vi "Release.vi"(8 "error in (no error)":errorcluster, 11 "Panel Registry in":refnum<class "Panel Registry.lvclass">) -> (0 "error out":errorcluster)   [LabVIEW 2023, in "Panel Actor.lvlib" / "Panel.lvlib" / "Panel Registry.lvclass"]
doc: "Releases a Panel Registry.\n\n----\nPlease see the following web address for additional documentation and tutorial information:\nhttp://www.mooregoodideas.com/mgi-panel-manager/\n\nAuthor: Derek Trepanier\n\nCopyright (c) 2018, Moore Good Ideas, Inc.\n\nAll rights reserved.\n\nRedistribution and use in source and binary forms, with or without modification, are permitted provided that the following conditions are met:\n\n * Redistributions of source code must retain the above copyright notice, this list of conditions and the following disclaimer.\n * Redistributions in binary form must reproduce the above copyright notice, this list of conditions and the following disclaimer in the documentation and/or other materials provided with the distribution.\n * Neither the name of Moore Good Ideas, Inc. nor the names of its contributors may be used to endorse or promote products derived from this software without specific prior written permission.\n\nTHIS SOFTWARE IS PROVIDED BY THE COPYRIGHT HOLDERS AND CONTRIBUTORS \"AS IS\" AND ANY EXPRESS OR IMPLIED WARRANTIES, INCLUDING, BUT NOT LIMITED TO, THE IMPLIED WARRANTIES OF MERCHANTABILITY AND FITNESS FOR A PARTICULAR PURPOSE ARE DISCLAIMED. IN NO EVENT SHALL THE COPYRIGHT OWNER OR CONTRIBUTORS BE LIABLE FOR ANY DIRECT, INDIRECT, INCIDENTAL, SPECIAL, EXEMPLARY, OR CONSEQUENTIAL DAMAGES (INCLUDING, BUT NOT LIMITED TO, PROCUREMENT OF SUBSTITUTE GOODS OR SERVICES; LOSS OF USE, DATA, OR PROFITS; OR BUSINESS INTERRUPTION) HOWEVER CAUSED AND ON ANY THEORY OF LIABILITY, WHETHER IN CONTRACT, STRICT LIABILITY, OR TORT (INCLUDING NEGLIGENCE OR OTHERWISE) ARISING IN ANY WAY OUT OF THE USE OF THIS SOFTWARE, EVEN IF ADVISED OF THE POSSIBILITY OF SUCH DAMAGE."
uses:
  Panel Registry.lvclass
  Panel Registry.lvclass/Panel Registry.ctl
  Static.vi
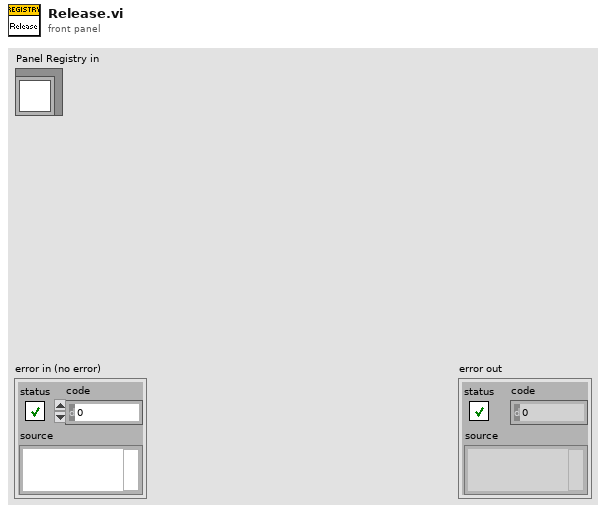
[diagram p1: front panel]
types:
  T1 = typedef "Semaphore RefNum" = refnum<k1>
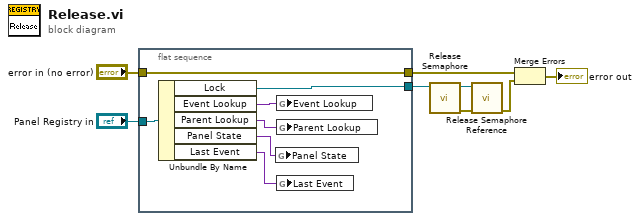
[diagram p0: block diagram]
diagram:
  n1 = flat-sequence {
    tunnel: "Panel Registry in" -> [w15]
    tunnel: [w14] -> w7
    tunnel: "error in (no error)" -> [w11]
    tunnel: [w11] -> w1
    frame #0 {
      n2 = Unbundle By Name(w15) -> ("Lock"=w14:T1, "Event Lookup"=w13:variant, "Parent Lookup"=w12:variant, "Panel State"=w10:variant, "Last Event"=w9:variant)
      n3 = global write "Static.vi" "Panel State"(w10) -> ()
      n4 = global write "Static.vi" "Event Lookup"(w13) -> ()
      n5 = global write "Static.vi" "Parent Lookup"(w12) -> ()
      n6 = global write "Static.vi" "Last Event"(w9) -> ()
    }
  }
  n7 = call <vilib>:"Release Semaphore.vi"("semaphore"=w7) -> ("error out"=w5:errorcluster, "semaphore out"=w6:T1)  [unwired: 5 in]
  n8 = call <vilib>:"Release Semaphore Reference.vi"("error in (no error)"=w5, "semaphore"=w6) -> ("error out"=w4:errorcluster)  [unwired: 8 in, 1 out]
  n9 = Merge Errors(w1, w4) -> (→"error out":errorcluster)
